vi "Test - Thermal Chamber Controller_DQMH - Update Set Point 1-setup.vi"(7 "test case ID":string, 8 "error in (no error)":errorcluster) -> (0 "error out":errorcluster, 2 "Temperature Set Point":dbl format="%#_13g")   [LabVIEW 2015]
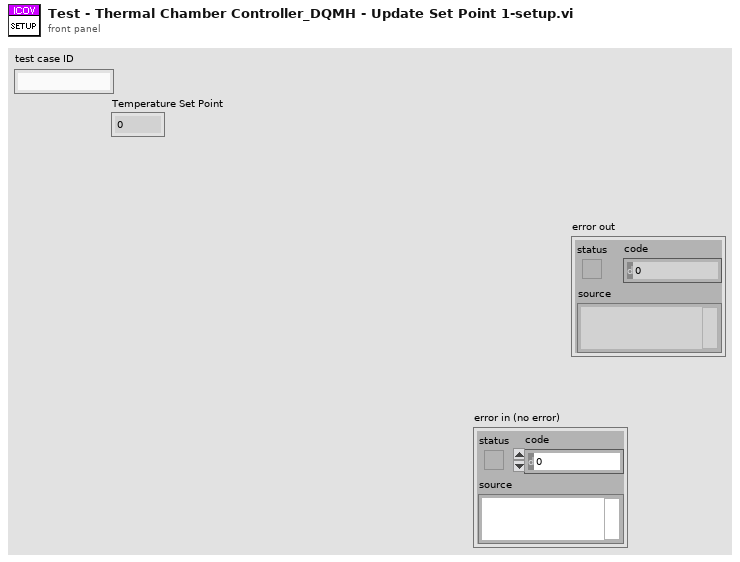
[diagram p1: front panel]
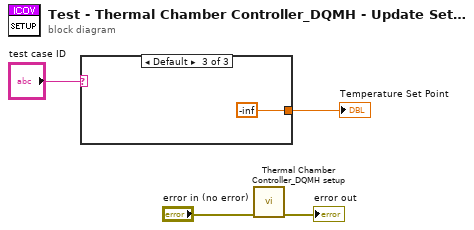
[diagram p0: block diagram]
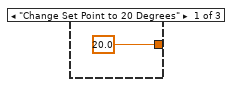
[diagram p2: hidden frame]
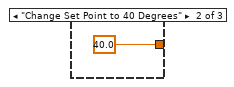
[diagram p3: hidden frame]
diagram:
  n1 = case shown="Default" "test case ID" {
    tunnel: [20.0 ("Temperature Set Point 2") 40.0 ("Temperature Set Point 2") -inf] -> w3
    frame "Change Set Point to 20 Degrees" {
    }
    frame "Change Set Point to 40 Degrees" {
    }
    frame Default {
    }
  }
  "Temperature Set Point" <- w3
  n2 = call "Thermal Chamber Controller_DQMH setup.vi"("error in (no error)"="error in (no error)") -> ("error out"=→"error out":errorcluster)  [unwired: 10 in]
